vi "Remote Client.vi"(5 "Port":u16=6341, 6 "timeout (ms) [500]":i32=500, 7 "address":string, 8 "error in (no error)":errorcluster, 9 "Data":variant, 10 "Command":string, 11 "RC Type":T1) -> (0 "error out":errorcluster, 1 "Data out":variant, 2 "Command out":string, 3 "RemoteControl out":refnum<class "RemoteControl.lvclass">)   [LabVIEW 2019, in "RemoteControl.lvclass"]
uses:
  RemoteControl.lvclass
  Typedefs/RC Com Type--enum.ctl
panel:
  # "Simple Client"
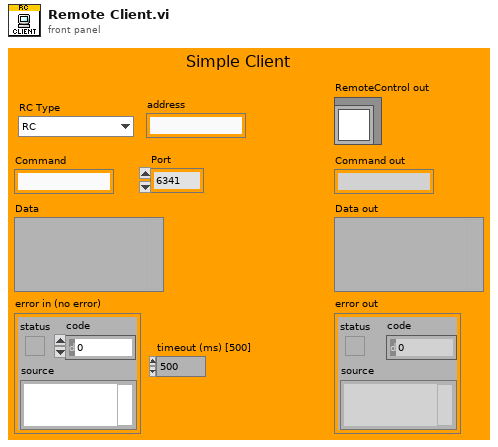
[diagram p1: front panel]
types:
  T1 = typedef "RemoteControl.lvclass/RC Com Type--enum.ctl" = enum16{"RC", "STM", "ZMQ"}
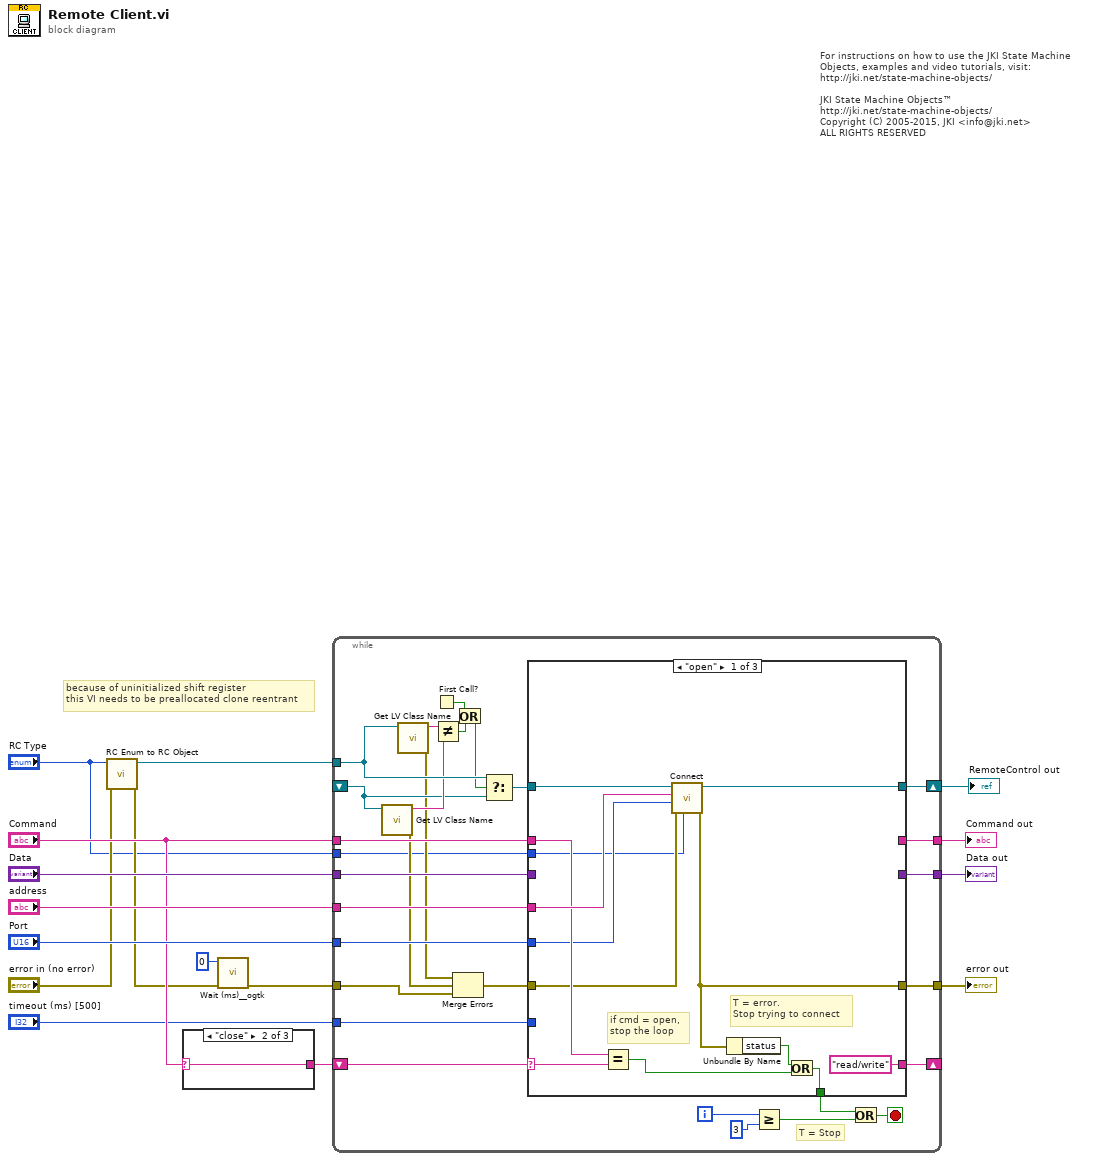
[diagram p0: block diagram]
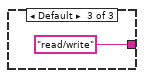
[diagram p3: hidden frame]
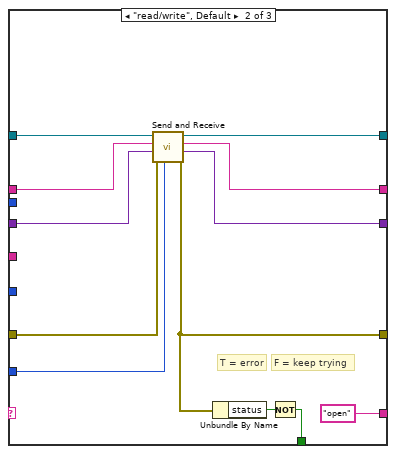
[diagram p4: hidden frame]
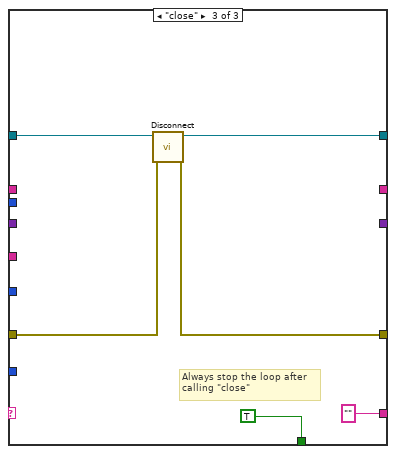
[diagram p5: hidden frame]
diagram:
  # "because of uninitialized shift register\nthis VI needs to be preallocated clone reentrant"
  # "For instructions on how to use the JKI State Machine Objects, examples and video tutorials, visit:\nhttp://jki.net/state-machine-objects/\n\nJKI State Machine Objects™\nhttp://jki.net/state-machine-objects/\nCopyright (C) 2005-2015, JKI <info@jki.net>\nALL RIGHTS RESERVED"
  n1 = call "RC Enum to RC Object.vi"("error in (no error)"="error in (no error)", "RC Type"="RC Type") -> ("error out"=w3:errorcluster, "RemoteControl out"=w5:refnum<class "RemoteControl.lvclass">)  [unwired: 8 in]
  n2 = case shown="\"close\"" "Command" {
    selector: "Command" -> [w17 w18 _]
    tunnel: [w17 w18 "read/write"] -> w8
    frame "open" {
    }
    frame "close" {
    }
    frame Default {
    }
  }
  n3 = call <userlib>:"Wait (ms)__ogtk.vi"("error in (no error)"=w3, "milliseconds to wait"=u32 0) -> ("error out"=w7:errorcluster)  [unwired: 8 in, 1 out]
  n4 = while {
    tunnel: "Port" -> [w46]
    tunnel: "address" -> [w45]
    shift-right: [w48] -> w15
    shift-left: _ -> [w23]
    shift-right: [w41] -> _
    shift-left: w8 -> [w34]
    tunnel: w5 -> [w33]
    tunnel: "Data" -> [w44]
    tunnel: [w42] -> w10
    tunnel: "Command" -> [w35]
    tunnel: [w43] -> w11
    tunnel: w7 -> [w25]
    tunnel: [w47] -> w16
    tunnel: "timeout (ms) [500]" -> [w21]
    tunnel: "RC Type" -> [w20]
    i -> [w40]
    stop <- w36 stop-if-true
    # "T = Stop"
    n5 = call <vilib>:"Get LV Class Name.vi"("object"=w23) -> ("error out"=w26:errorcluster, "class name"=w27:string)  [unwired: 9 in]
    n6 = call <vilib>:"Get LV Class Name.vi"("object"=w33) -> ("error out"=w22:errorcluster, "class name"=w32:string)  [unwired: 9 in]
    n7 = First Call?() -> (First Call?: T/F=w31:bool)
    n8 = Not Equal?(x=w32, y=w27) -> (x != y?=w30:bool)
    n9 = Merge Errors(w22, w26, w25) -> (w24:errorcluster)
    n10 = Or(x=w31, y=w30) -> (x .or. y?=w28:bool)
    n11 = Select(t=w33, s=w28, f=w23) -> (s? t:f=w29:refnum<class "RemoteControl.lvclass">)
    n12 = case shown="\"open\"" w34 {
      selector: w34 -> [w58 _ _]
      tunnel: [w60 w73 w79] -> w48
      tunnel: [w50 w67 w74] -> w47
      tunnel: w46 -> [w52 _ _]
      tunnel: w24 -> [w53 w68 w75]
      tunnel: w45 -> [w61 _ _]
      tunnel: w44 -> [_ w62 _]
      tunnel: w35 -> [w57 w65 _]
      tunnel: [_ w66 _] -> w43
      tunnel: [_ w72 _] -> w42
      tunnel: ["read/write" "open" ""] -> w41
      tunnel: [w55 w69 TRUE] -> w38
      tunnel: w29 -> [w51 w64 w76]
      tunnel: w21 -> [_ w63 _]
      tunnel: w20 -> [w49 _ _]
      frame "open" {
        # "if cmd = open,\nstop the loop"
        # "T = error.\nStop trying to connect"
        n13 = Equal?(x=w57, y=w58) -> (x = y?=w56:bool)
        n14 = call "Connect.vi"("RC Type"=w49, "error in (no error)"=w53, "Port"=w52, "address"=w61, "RemoteControl in"=w51) -> ("error out"=w50:errorcluster, "RemoteControl out"=w60:refnum<class "RemoteControl.lvclass">)  [unwired: 5 in]
        n15 = Unbundle By Name(w50) -> ("status"=w54:bool)
        n16 = Or(x=w54, y=w56) -> (x .or. y?=w55:bool)
      }
      frame "read/write", Default {
        # "F = keep trying"
        # "T = error"
        n17 = call "Send and Receive.vi"("timeout (ms) [500]"=w63, "error in (no error)"=w68, "Data"=w62, "Command"=w65, "RemoteControl in"=w64) -> ("error out"=w67:errorcluster, "Data out"=w72:variant, "Command out"=w66:string, "RemoteControl out"=w73:refnum<class "RemoteControl.lvclass">)  [unwired: 3 in]
        n18 = Unbundle By Name(w67) -> ("status"=w70:bool)
        n19 = Not(x=w70) -> (.not. x?=w69:bool)
      }
      frame "close" {
        # "Always stop the loop after\ncalling \"close\""
        n20 = call "Disconnect.vi"("error in (no error)"=w75, "RemoteControl in"=w76) -> ("error out"=w74:errorcluster, "RemoteControl out"=w79:refnum<class "RemoteControl.lvclass">)  [unwired: 8 in]
      }
    }
    n21 = Greater Or Equal?(x=w40, y=3) -> (x >= y?=w37:bool)
    n22 = Or(x=w38, y=w37) -> (x .or. y?=w36:bool)
  }
  "RemoteControl out" <- w15
  "error out" <- w16
  "Data out" <- w10
  "Command out" <- w11
